vi "Authorization Save Site Key.vi"(8 "error in (no error)":errorcluster, 11 "Spartan License.xml":string) -> (0 "error out":errorcluster)   [LabVIEW 2011]
doc: "The SaveSiteKey() function is used to save to a file the site key issued to the user. The key is checked first before it is saved.\n\nIf the program detects it is not authorized via the GetAuthorization() function, it must, at minimum, show the program's site code and allow the user to enter a site key."
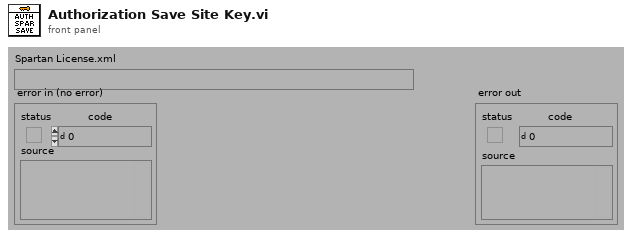
[diagram p1: front panel]
types:
  T1 = enum16{"open", "replace", "create", "open or create", "replace or create", "replace or create with confirmation"}
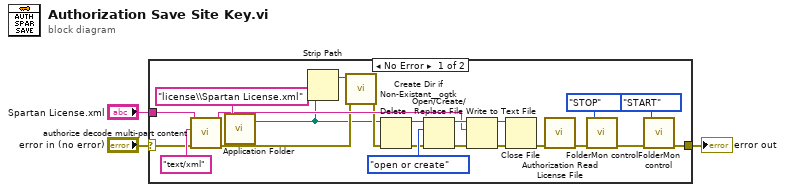
[diagram p0: block diagram]
diagram:
  n1 = case shown="No Error" "error in (no error)" {
    selector: "error in (no error)" -> [w17 w25]
    tunnel: [w8 w25] -> w3
    tunnel: "Spartan License.xml" -> [w16 _]
    frame No Error {
      n2 = call "authorize decode multi-part content.vi"("error in (no error)"=w17, "Valid Content-Type: (\"text/xml\")"="text/xml" ("Relative Path (\"\" - Folder)"), "Multi-Part Content (\"\")"=w16) -> ("error out"=w7:errorcluster, "Content"=w15:string)  [unwired: 7 in]
      n3 = call "Application Folder.vi"("Relative Path (\"\" - Folder)"="license\\Spartan License.xml" ("regular expression")) -> ("Application Folder"=w5:path)  [unwired: 2 in]
      n4 = Strip Path(path=w5) -> (stripped path=w4:path)  [unwired: 1 out]
      n5 = call "Create Dir if Non-Existant__ogtk.vi"("error in (no error)"=w7, "Directory Path"=w4) -> ("error out"=w6:errorcluster)  [unwired: 7 in, 2 out]
      n6 = Delete(path (use dialog)=w5, error in=w6) -> (deleted path=w13:path)  [unwired: 3 in, 2 out]
      n7 = Open/Create/Replace File(file path (use dialog)=w13, error in=w6, operation (0:open)=T1."open or create") -> (refnum out=w21:refnum<file>, error out=w24:errorcluster)  [unwired: 3 in, 1 out]
      n8 = Write to Text File(file (use dialog)=w21, text=w15, error in=w24) -> (refnum out=w20:refnum<file>, error out=w23:errorcluster)  [unwired: 1 in, 1 out]
      n9 = Close File(refnum=w20, error in=w23) -> (error out=w19:errorcluster)  [unwired: 1 out]
      n10 = call "Authorization Read License File.vi"("error in (no error)"=w19) -> ("error out"=w11:errorcluster)  [unwired: 9 in, 1 out]
      n11 = call "FolderMon control.vi"("error in (no error)"=w11, "Action (START)"=enum16{"START", "STOP"}."STOP") -> ("error out"=w9:errorcluster)  [unwired: 1 in, 4 out]
      n12 = call "FolderMon control.vi"("error in (no error)"=w9, "Action (START)"=enum16{"START", "STOP"}."START") -> ("error out"=w8:errorcluster)  [unwired: 1 in, 4 out]
    }
    frame Error {
    }
  }
  "error out" <- w3
